vi "CAN Set Value.vi"(7 "BufferLength":u32, 8 "error in (no error)":errorcluster caption="错误输入（无错误）", 9 "Buffer":u32, 10 "Parameter":u8, 11 "Channel":u8) -> (0 "error out":errorcluster caption="错误输出", 1 "Buffer out":u32, 3 "function return":u32)   [LabVIEW 2021]
doc: "TPCANStatus __stdcall CAN_SetValue(\n TPCANHandle Channel,\n TPCANParameter Parameter,\n void* Buffer,\n DWORD BufferLength);"
uses:
  PCANBasic.dll
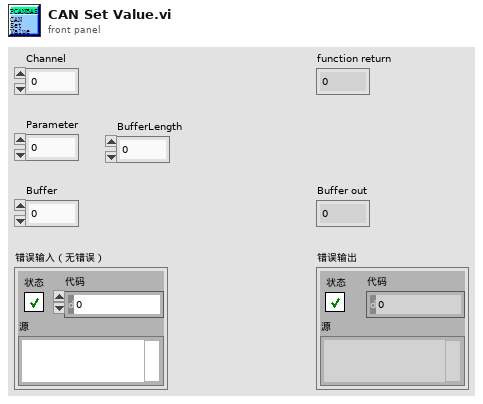
[diagram p1: front panel]
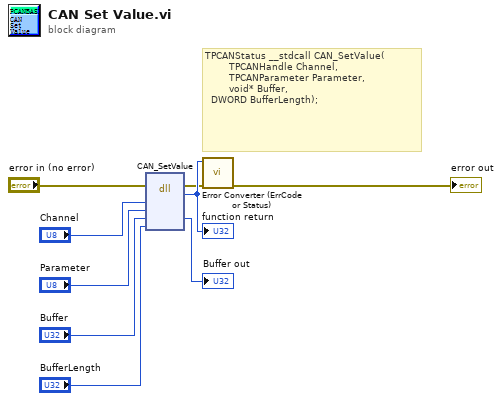
[diagram p0: block diagram]
diagram:
  # "TPCANStatus __stdcall CAN_SetValue(\n        TPCANHandle Channel,\n        TPCANParameter Parameter,\n        void* Buffer,\n\t\tDWORD BufferLength);"
  n1 = dll-call lib="D:/ON LINE WORK/LabVIEW/PCAN/PCAN 1.6(2021)/PCANBasic.*" fn="CAN_SetValue"(error in="error in (no error)", "Channel"="Channel", "Parameter"="Parameter", "Buffer"="Buffer", "BufferLength"="BufferLength") -> (error out=w2:errorcluster, "返回类型"=w9:u32, "Buffer"=→"Buffer out":u32)  [unwired: 5 in, 1 out]
  "function return" <- w9
  n2 = call "Error Converter (ErrCode or Status).vi"("error in (no error)"=w2, "error code"=w9) -> ("error out"=→"error out":errorcluster)  [unwired: 9 in]
